vi "create 4 corner roi.vi"(8 "error in (no error)":errorcluster, 11 "Refnum in":T1) -> (0 "error out":errorcluster, 3 "ROI Descriptor":T2 {"Contours"."Type" items=["No Selection", "Point", "Line", "Rectangle", "Oval", "Polygon", "Freehand Region", "Annulus", "Unused2", "Unused3", "Broken Line", "Freehand Line", "Rotated Rectangle"]})   [LabVIEW 2020]
uses:
  IMAQ Image.ctl
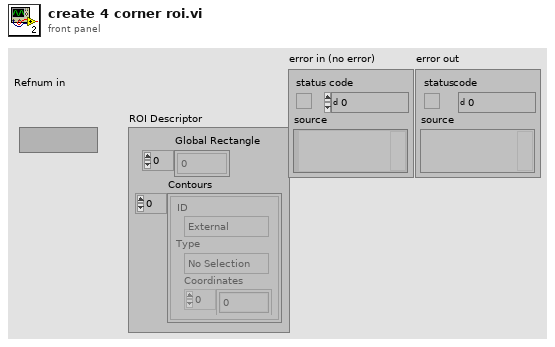
[diagram p1: front panel]
types:
  T1 = typedef "IMAQ Image.ctl" = refnum<image>
  T2 = typedef "ROI Descriptor" = cluster{"Global Rectangle":i32[], "Contours":cluster{"ID":enum32{"External", "Internal"}, "Type":u32, "Coordinates":i32[]}[]}
  T3 = cluster{"ID":enum32{"External", "Internal"}, "Type":u32, "Coordinates":i32[]}[]
  T4 = cluster{"ID":enum32{"External", "Internal"}, "Type":u32, "Coordinates":i32[]}
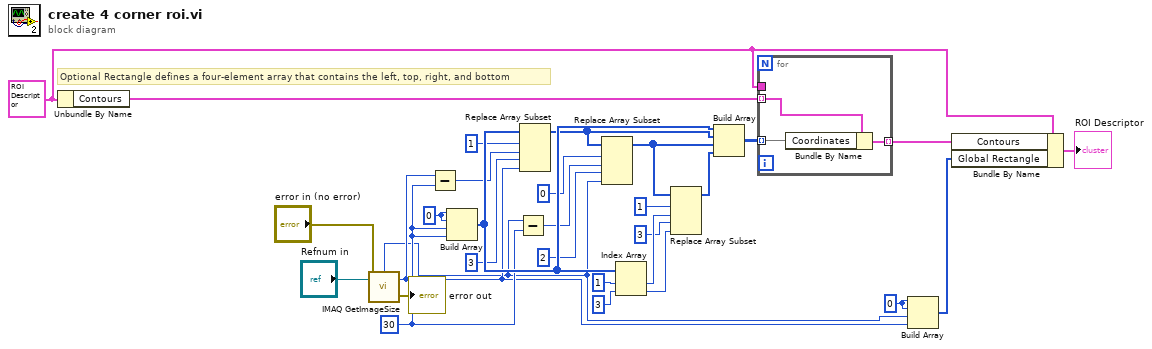
[diagram p0: block diagram]
diagram:
  w21 = T2 {"Global Rectangle"=[0, 0, 0, 0], "Contours"=[{"ID"=enum."External", "Type"=3, "Coordinates"=[]}, {"ID"=enum."External", "Type"=3, "Coordinates"=[]}, {"ID"=enum."External", "Type"=3, "Coordinates"=[]}, {"ID"=enum."External", "Type"=3, "Coordinates"=[]}]} ("ROI Descriptor")
  w28 = 0 ("y")
  w24 = 0 ("y")
  w29 = 30 ("y")
  # "Optional Rectangle defines a four-element array that contains the left, top, right, and bottom"
  n1 = Unbundle By Name(w21) -> ("Contours"=w20:T3)
  n2 = call "IMAQ GetImageSize"("Image"="Refnum in", "error in (no error)"="error in (no error)") -> ("Y Resolution"=w26:i32, "X Resolution"=w25:i32, "error out"=→"error out":errorcluster)  [unwired: 2 in]
  n3 = Subtract(x=w26, y=w29) -> (x-y=w6:i32)
  n4 = Build Array(w28, w28, w29, w29) -> (w30:i32[])
  n5 = Subtract(x=w25, y=w29) -> (x-y=w9:i32)
  n6 = Replace Array Subset(array=w30, new element #1=w6, index #1=1 ("index"), new element #2=w26, index #2=3 ("index")) -> (w16:i32[])
  n7 = Replace Array Subset(array=w16, new element #1=w9, index #1=0 ("index"), new element #2=w25, index #2=2 ("index")) -> (w17:i32[])
  n8 = Index Array(array=w30, index #1=1 ("index"), index #2=3 ("index")) -> (element #1=w14:i32, element #2=w15:i32)
  n9 = Replace Array Subset(array=w17, new element #1=w14, index #1=1 ("index"), new element #2=w15, index #2=3 ("index")) -> (w18:i32[])
  n10 = Build Array(w30, w16, w17, w18) -> (w19:i32[][])
  n11 = for {
    tunnel: w21 -> [_]
    tunnel: w19 -> [w32] mode=indexing
    tunnel: [w31] -> w22 mode=indexing
    tunnel: w20 -> [w33] mode=indexing
    n12 = Bundle By Name(cluster=w33, "Coordinates"=w32) -> (w31:T4)
  }
  n13 = Build Array(w24, w24, w25, w26) -> (w27:i32[])
  n14 = Bundle By Name(cluster=w21, "Contours"=w22, "Global Rectangle"=w27) -> (→"ROI Descriptor":T2)
